vi "Initialize Generate.vi"(8 "error in (no error)":errorcluster, 10 "PCL (usec)":u32, 11 "OnCompile Variables":T9={"XNET Settings"={"Database"="", "Cluster"="", "Port"="", "Baud rate [Bd]"=500000, "Termination"=1, "CAN I/O Mode"=0, "FD Baud rate [Bd]"=500000, "Priority"=100, "Use Legacy"=FALSE}, "Frames"=[], "986x Support"={"Enable"=FALSE, "RIO Device"="", "Bitfile"=path ""}} {"XNET Settings"."CAN I/O Mode" items=["CAN 2.0", "CAN FD", "CAN FD+BRS"]; "XNET Settings"."Termination" items=["Off", "On"]; "Frames"."Protection Configurations"."CRC Channels"."Data Type" items=["Signed", "Unsigned", "IEEE Float"]}) -> (0 "error out":errorcluster, 3 "RT Configuration":T1={"Priority"=100, "CAN Session"="", "Frame Count"=0, "Frames"=[], "FPGA Session"=0} {"Frames"."Protection Configurations"."CRC Channels"."Data Type" items=["Signed", "Unsigned", "IEEE Float"]})   [LabVIEW 2015, in "Protection and Rolling Counter Addon Engine.lvlib"]
uses:
  Protection and Rolling Counter Addon Engine.lvlib
  Shared/Types/Exported.OnCompile.ctl
  Shared/Types/XNET Settings.ctl
  Shared/Types/Exported Frame Settings.ctl
  Shared/Types/Exported Frame Type.ctl
  Shared/Types/Exported Protection Settings.ctl
  Shared/Types/Protection Type.ctl
  Shared/Types/InputChannelConfiguration.ctl
  Shared/Types/Exported Counter Settings.ctl
  Shared/Types/Event Trigger Type.ctl
  Shared/Types/986x.ctl
  Types/RT Async Engine Variables.ctl
  Types/RT Frame Settings.ctl
  Types/RT Protection Configuration.ctl
  Types/RT Counter Settings.ctl
  <vilib>/xnet/xnet.llb/XNET Create Session (Frame Output Stream).vi
  <vilib>/xnet/xnet.llb/XNET Create Session (Conversion).vi
  Shared/Protection and Rolling Counter Addon Shared.lvlib
  <resource>/objmgr/xnet.rc
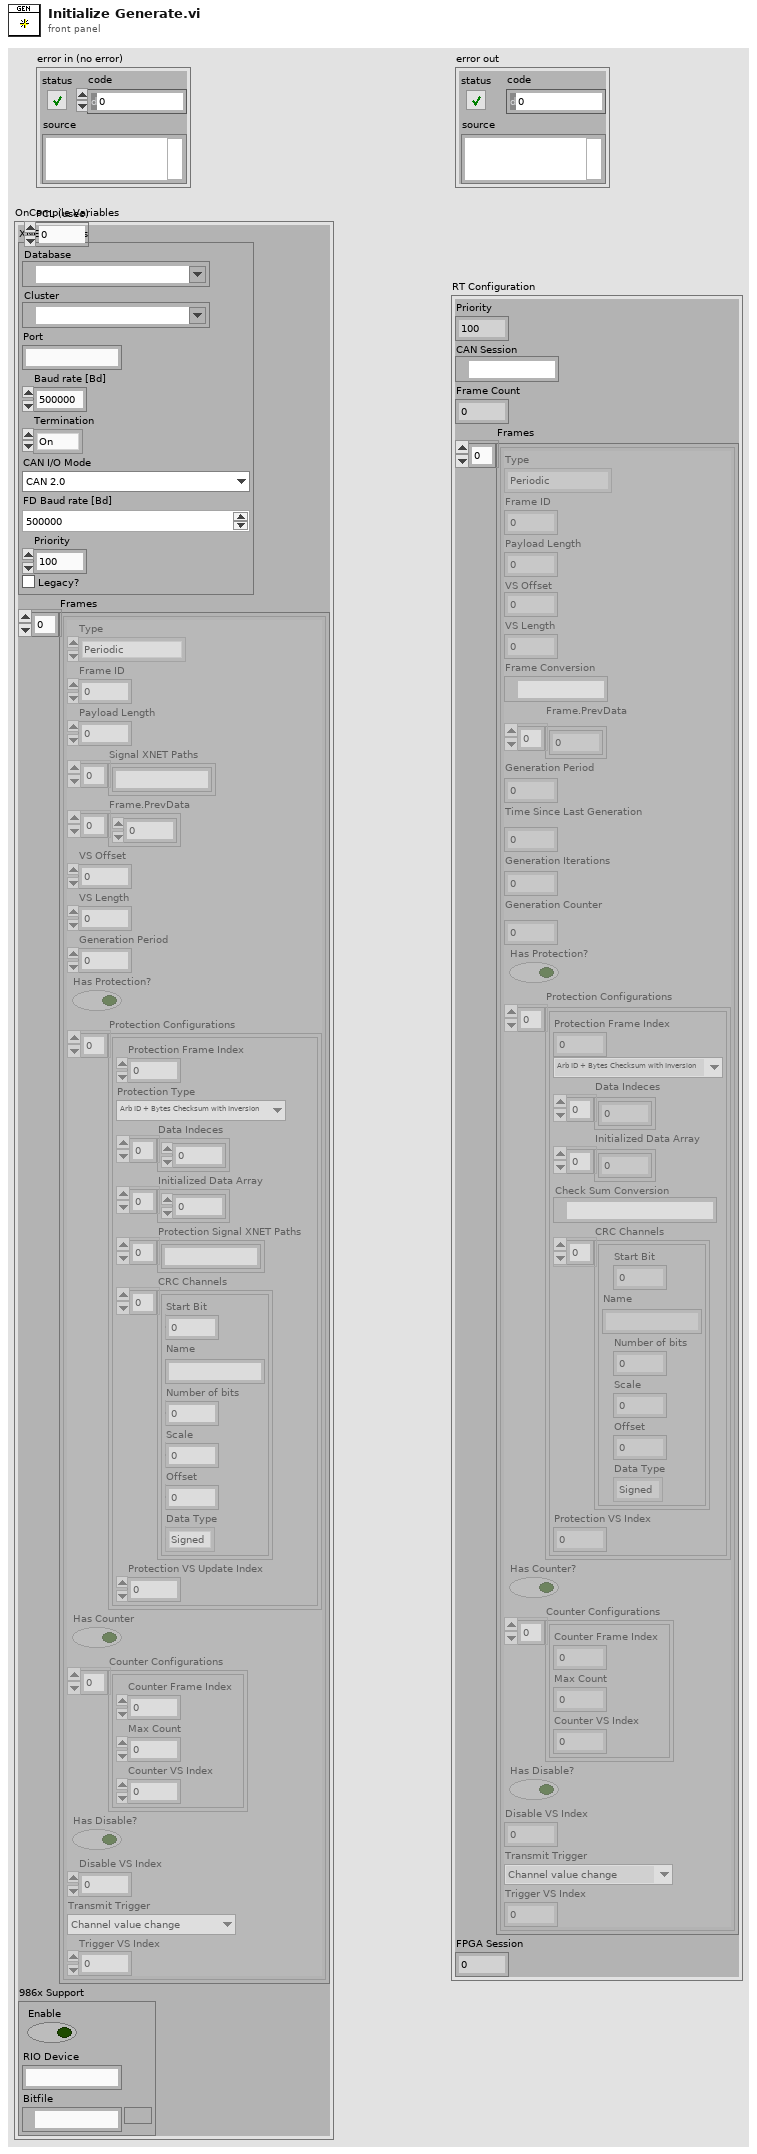
[diagram p1: front panel]
types:
  T1 = typedef "Protection and Rolling Counter Addon Engine.lvlib/RT Async Engine Variables.ctl" = cluster{"Priority":i32, "CAN Session":refnum<k21>, "Frame Count":i32, "Frames":T2[], "FPGA Session":u32}
  T2 = typedef "Protection and Rolling Counter Addon Engine.lvlib/RT Frame Settings.ctl" = cluster{"Type":T3, "Frame ID":u32, "Payload Length":u32, "VS Offset":i32, "VS Length":i32, "Frame Conversion":refnum<k21>, "Frame.PrevData":dbl[], "Generation Period":u32, "Time Since Last Generation":u32, "Generation Iterations":u32, "Generation Counter":u32, "Has Protection?":bool, "Protection Configurations":T4[], "Has Counter?":bool, "Counter Configurations":T7[], "Has Disable?":bool, "Disable VS Index":i32, "Transmit Trigger":T8, "Trigger VS Index":i32}
  T3 = typedef "Protection and Rolling Counter Addon Shared.lvlib/Exported Frame Type.ctl" = enum16{"Periodic", "Event", "Periodic/Event"}
  T4 = typedef "Protection and Rolling Counter Addon Engine.lvlib/RT Protection Configuration.ctl" = cluster{"Protection Frame Index":i32, "Protection Type":T5, "Data Indeces":i32[], "Initialized Data Array":dbl[], "Check Sum Conversion":refnum<k21>, "CRC Channels":T6[], "Protection VS Index":i32}
  T5 = typedef "Protection and Rolling Counter Addon Shared.lvlib/Protection Type.ctl" = enum16{"Arb ID + Bytes Checksum with Inversion", "Arb ID + Bytes CRC with Inversion", "Reversed Raw Signal Checksum with Inversion"}
  T6 = typedef "Protection and Rolling Counter Addon Shared.lvlib/InputChannelConfiguration.ctl" = cluster{"Start Bit":i32, "Name":string, "Number of bits":i32, "Scale":dbl, "Offset":dbl, "Data Type":u32}
  T7 = typedef "Protection and Rolling Counter Addon Engine.lvlib/RT Counter Settings.ctl" = cluster{"Counter Frame Index":i32, "Max Count":dbl, "Counter VS Index":i32}
  T8 = typedef "Protection and Rolling Counter Addon Shared.lvlib/Event Trigger Type.ctl" = enum16{"Channel value change", "Trigger channel (not zero)", "Channel value change or trigger channel (not zero)", "Trigger channel (any value change)", "Channel value change or trigger channel (any value change)"}
  T9 = typedef "Protection and Rolling Counter Addon Shared.lvlib/Exported.OnCompile.ctl" = cluster{"XNET Settings":T10, "Frames":T11[], "986x Support":T14}
  T10 = typedef "Protection and Rolling Counter Addon Shared.lvlib/XNET Settings.ctl" = cluster{"Database":refnum<k21>, "Cluster":refnum<k21>, "Port":string, "Baud rate [Bd]":u64, "Termination":u32, "CAN I/O Mode":u32, "FD Baud rate [Bd]":u64, "Priority":i32, "Use Legacy":bool}
  T11 = typedef "Protection and Rolling Counter Addon Shared.lvlib/Exported Frame Settings.ctl" = cluster{"Type":T3, "Frame ID":u32, "Payload Length":u32, "Signal XNET Paths":string[], "Frame.PrevData":dbl[], "VS Offset":i32, "VS Length":i32, "Generation Period":u32, "Has Protection?":bool, "Protection Configurations":T12[], "Has Counter":bool, "Counter Configurations":T13[], "Has Disable?":bool, "Disable VS Index":i32, "Transmit Trigger":T8, "Trigger VS Index":i32}
  T12 = typedef "Protection and Rolling Counter Addon Shared.lvlib/Exported Protection Settings.ctl" = cluster{"Protection Frame Index":i32, "Protection Type":T5, "Data Indeces":i32[], "Initialized Data Array":dbl[], "Protection Signal XNET Paths":string[], "CRC Channels":T6[], "Protection VS Update Index":i32}
  T13 = typedef "Protection and Rolling Counter Addon Shared.lvlib/Exported Counter Settings.ctl" = cluster{"Counter Frame Index":i32, "Max Count":dbl, "Counter VS Index":i32}
  T14 = typedef "Protection and Rolling Counter Addon Shared.lvlib/986x.ctl" = cluster{"Enable":bool, "RIO Device":string, "Bitfile":path}
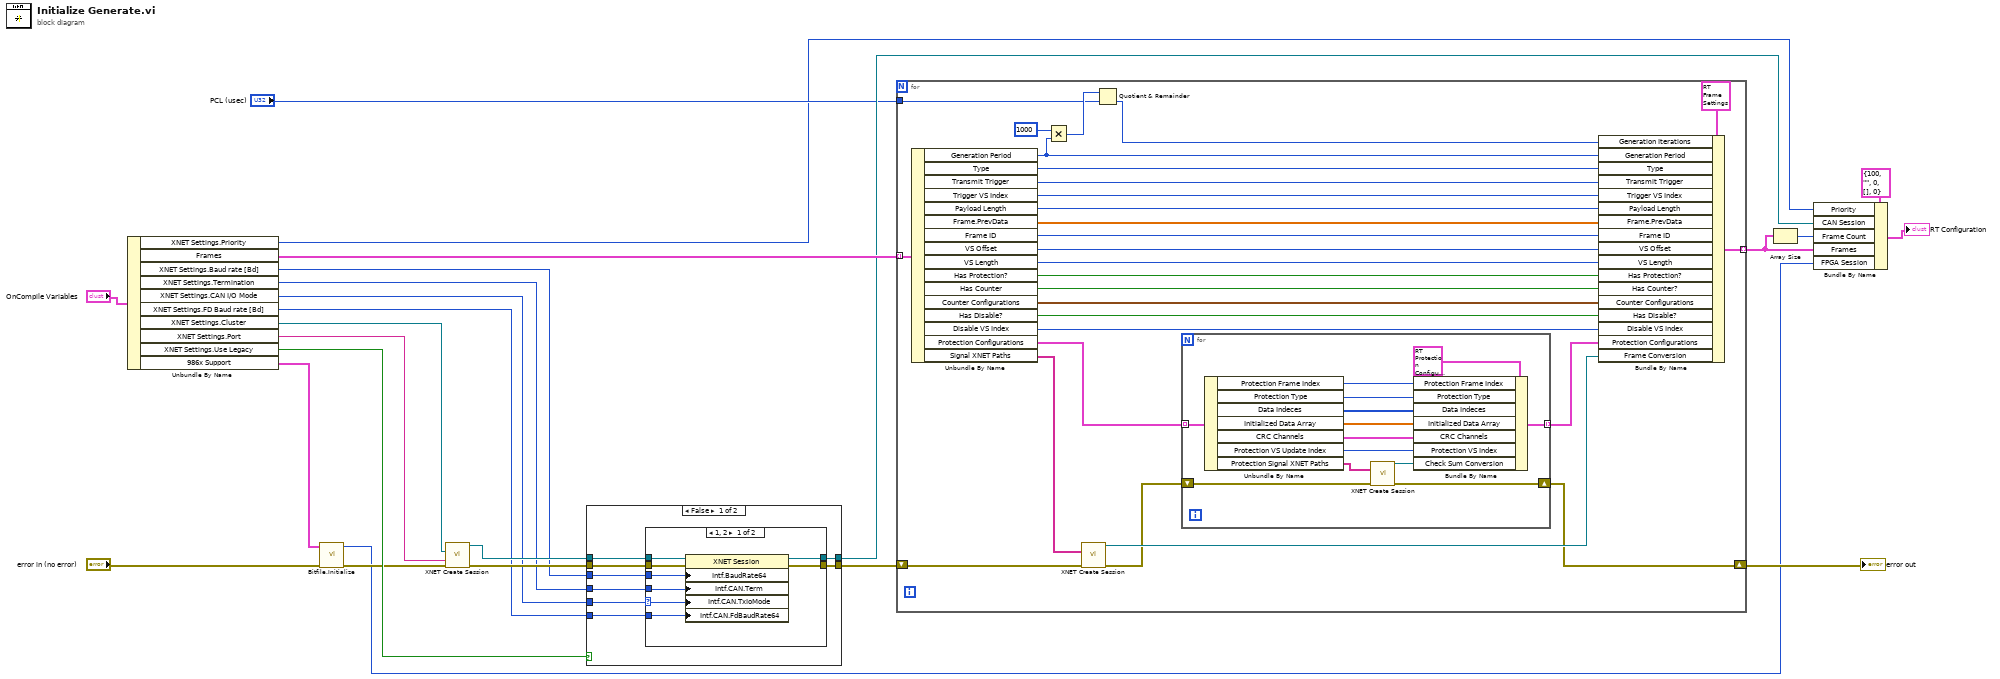
[diagram p0: block diagram]
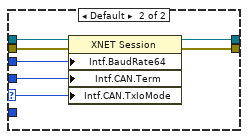
[diagram p2: hidden frame]
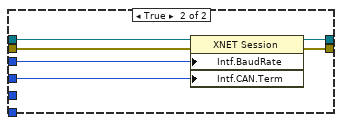
[diagram p3: hidden frame]
diagram:
  n1 = Unbundle By Name("OnCompile Variables") -> ("XNET Settings.Priority"=w6:i32, "Frames"=w23:T11[], "XNET Settings.Baud rate [Bd]"=w11:u64, "XNET Settings.Termination"=w12:u32, "XNET Settings.CAN I/O Mode"=w13:u32, "XNET Settings.FD Baud rate [Bd]"=w14:u64, "XNET Settings.Cluster"=w16:refnum<k21>, "XNET Settings.Port"=w15:string, "XNET Settings.Use Legacy"=w5:bool, "986x Support"=w2:T14)
  n2 = call "Bitfile.Initialize.vi"("error in (no error)"="error in (no error)", "FPGA Bitfile Settings"=w2) -> ("error out"=w3:errorcluster, "FPGA Session"=w1:u32)  [unwired: 8 in]
  n3 = call-poly <vilib>:"XNET Create Session.vi"("cluster (:memory:)"=w16, "interface"=w15, "error in (no error)"=w3) -> ("session out"=w18:refnum<k21>, "error out"=w19:errorcluster)  [unwired: 11 in]
  n4 = case shown="False" w5 {
    tunnel: w19 -> [w32 w53]
    tunnel: w18 -> [w31 w52]
    tunnel: [w30 w51] -> w17
    tunnel: w14 -> [w29 _]
    tunnel: w13 -> [w25 _]
    tunnel: w12 -> [w28 w48]
    tunnel: w11 -> [w27 w49]
    tunnel: [w26 w50] -> w10
    frame False {
      n5 = case shown="1, 2" w25 {
        selector: w25 -> [w33 w41]
        tunnel: w32 -> [w40 w47]
        tunnel: w31 -> [w39 w46]
        tunnel: [w38 w45] -> w30
        tunnel: w29 -> [w37 _]
        tunnel: w28 -> [w36 w44]
        tunnel: w27 -> [w35 w43]
        tunnel: [w34 w42] -> w26
        frame 1, 2 {
          n6 = property class="XNET Session"(reference=w39, error in=w40, "Intf.BaudRate64"=w35, "Intf.CAN.Term"=w36, "Intf.CAN.TxIoMode"=w33, "Intf.CAN.FdBaudRate64"=w37) -> (reference out=w34:refnum<k21>, error out=w38:errorcluster)
        }
        frame Default {
          n7 = property class="XNET Session"(reference=w46, error in=w47, "Intf.BaudRate64"=w43, "Intf.CAN.Term"=w44, "Intf.CAN.TxIoMode"=w41) -> (reference out=w42:refnum<k21>, error out=w45:errorcluster)
        }
      }
    }
    frame True {
      n8 = property class="XNET Session"(reference=w52, error in=w53, "Intf.BaudRate"=w49, "Intf.CAN.Term"=w48) -> (reference out=w50:refnum<k21>, error out=w51:errorcluster)
    }
  }
  n9 = for {
    shift-right: [w66] -> w22
    shift-left: w17 -> [w79]
    tunnel: w23 -> [w81] mode=indexing
    tunnel: [w65] -> w7 mode=indexing
    tunnel: "PCL (usec)" -> [w60]
    n10 = Unbundle By Name(w81) -> ("Generation Period"=w59:u32, "Type"=w54:T3, "Transmit Trigger"=w55:T8, "Trigger VS Index"=w56:i32, "Payload Length"=w57:u32, "Frame.PrevData"=w63:dbl[], "Frame ID"=w77:u32, "VS Offset"=w76:i32, "VS Length"=w75:i32, "Has Protection?"=w74:bool, "Has Counter"=w73:bool, "Counter Configurations"=w72:T13[], "Has Disable?"=w71:bool, "Disable VS Index"=w70:i32, "Protection Configurations"=w69:T12[], "Signal XNET Paths"=w80:string[])
    n11 = Multiply(x=u32 1000, y=w59) -> (x*y=w61:u32)
    n12 = call-poly <vilib>:"XNET Create Session.vi"("signal list"=w80, "error in (no error)"=w79) -> ("session out"=w78:refnum<k21>, "error out"=w67:errorcluster)  [unwired: 12 out]
    n13 = Quotient & Remainder(x=w61, y=w60) -> (floor(x/y)=w58:u32)  [unwired: 1 out]
    n14 = for {
      tunnel: w69 -> [w94] mode=indexing
      tunnel: [w84] -> w68 mode=indexing
      shift-right: [w82] -> w66
      shift-left: w67 -> [w83]
      n15 = Unbundle By Name(w94) -> ("Protection Frame Index"=w92:i32, "Protection Type"=w91:T5, "Data Indeces"=w90:i32[], "Initialized Data Array"=w89:dbl[], "CRC Channels"=w88:T6[], "Protection VS Update Index"=w87:i32, "Protection Signal XNET Paths"=w86:string[])
      n16 = call-poly <vilib>:"XNET Create Session.vi"("signal list"=w86, "error in (no error)"=w83) -> ("session out"=w85:refnum<k21>, "error out"=w82:errorcluster)  [unwired: 12 out]
      n17 = Bundle By Name(cluster=T4 {"Protection Frame Index"=0, "Protection Type"=enum."Arb ID + Bytes Checksum with Inversion", "Data Indeces"=[], "Initialized Data Array"=[], "Check Sum Conversion"="", "CRC Channels"=[], "Protection VS Index"=0} ("Cluster"), "Protection Frame Index"=w92, "Protection Type"=w91, "Data Indeces"=w90, "Initialized Data Array"=w89, "CRC Channels"=w88, "Protection VS Index"=w87, "Check Sum Conversion"=w85) -> (w84:T4)
    }
    n18 = Bundle By Name(cluster=T2 {"Type"=enum."Periodic", "Frame ID"=0, "Payload Length"=0, "VS Offset"=0, "VS Length"=0, "Frame Conversion"="", "Frame.PrevData"=[], "Generation Period"=0, "Time Since Last Generation"=0, "Generation Iterations"=0, "Generation Counter"=0, "Has Protection?"=FALSE, "Protection Configurations"=[], "Has Counter?"=FALSE, "Counter Configurations"=[], "Has Disable?"=FALSE, "Disable VS Index"=0, "Transmit Trigger"=enum."Channel value change", "Trigger VS Index"=0} ("Frame Settings"), "Generation Iterations"=w58, "Generation Period"=w59, "Type"=w54, "Transmit Trigger"=w55, "Trigger VS Index"=w56, "Payload Length"=w57, "Frame.PrevData"=w63, "Frame ID"=w77, "VS Offset"=w76, "VS Length"=w75, "Has Protection?"=w74, "Has Counter?"=w73, "Counter Configurations"=w72, "Has Disable?"=w71, "Disable VS Index"=w70, "Protection Configurations"=w68, "Frame Conversion"=w78) -> (w65:T2)
  }
  "error out" <- w22
  n19 = Array Size(array=w7) -> (size(s)=w8:i32)
  n20 = Bundle By Name(cluster=T1 {"Priority"=100, "CAN Session"="", "Frame Count"=0, "Frames"=[], "FPGA Session"=0} ("RT Configuration"), "Priority"=w6, "CAN Session"=w10, "Frame Count"=w8, "Frames"=w7, "FPGA Session"=w1) -> (→"RT Configuration":T1)
